vi "RunAcquisition.vi"(8 "error in (no error)":errorcluster, 11 "NIScope in":refnum<class "NIScope.lvclass">) -> (0 "error out":errorcluster, 1 "output cluster":T1, 2 "Waveforms":T3[](array[typedef]), 3 "NIScope out":refnum<class "NIScope.lvclass">)   [LabVIEW 2018, in "ScopePlugins.lvlib" / "NIScope.lvclass"]
doc: "Retrieves data from the instrument(s)."
uses:
  NIScope.lvclass
  F:/Projects/ICDAS/NistPluggableModules/Scope/ScopePlugins/ScopePluginBaseClass/ScopePluginsBase.lvclass
  ScopeShared/Waveform.ctl
  ScopeShared/ScopeData.ctl
  ScopePluginBaseClass/ScopePluginsBase.lvclass/ScopePluginsBase.ctl
  ScopePluginBaseClass/Accessors/Read Channels.vi
  <instrlib>/niScope/Acquire/Fetch/niScope Multi Fetch Cluster.vi
  ScopePlugins.lvlib
  ScopeShared/ScopeShared.lvlib
panel:
  out "Waveform Graph":T2(graph)
  out "Absolute":dbl[](array[numeric])
  out "Relative":dbl[](array[numeric])
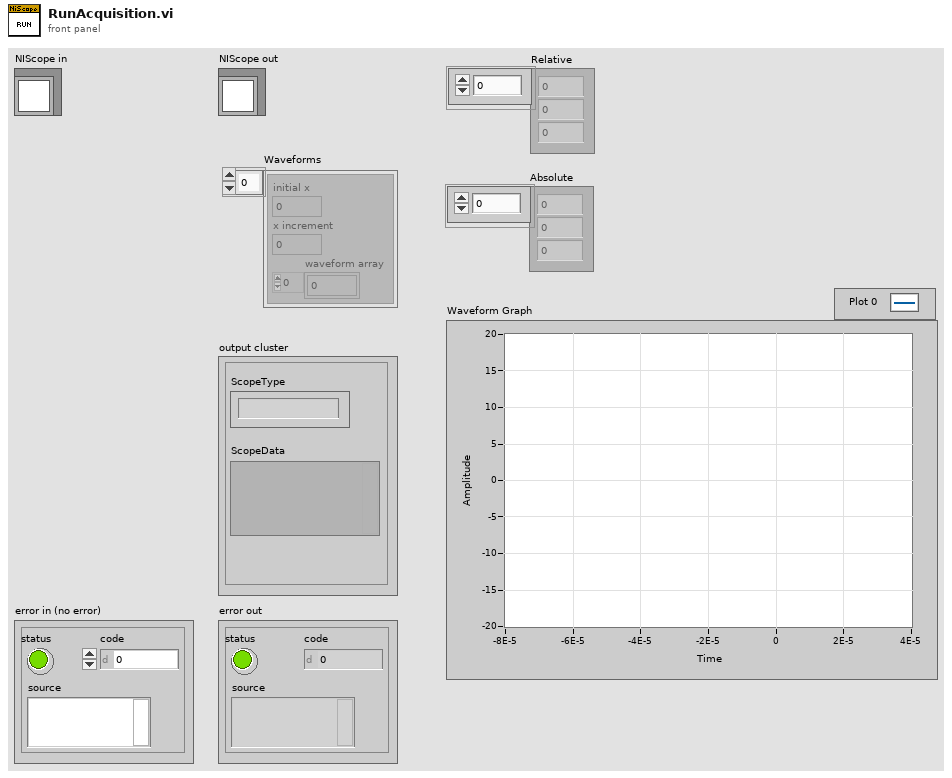
[diagram p1: front panel]
types:
  T1 = typedef "ScopeShared.lvlib/ScopeData.ctl" = cluster{"ScopeType":string, "ScopeData":variant}
  T2 = cluster{"relativeInitialX":dbl, "xIncrement":dbl, "wfm":dbl[]}[]
  T3 = typedef "ScopeShared.lvlib/Waveform.ctl" = cluster{"initial x":dbl, "x increment":dbl, "waveform array":dbl[]}
  T4 = typedef "ScopePlugins.lvlib/ScopePluginsBase.lvclass/InitializationSettings.ctl" = cluster{"Reset":bool, "IdQuery":bool, "AutoConfig":bool, "Options String":string, "Synchronize":bool}
  T5 = typedef "ScopePlugins.lvlib/ScopePluginsBase.lvclass/HorizontalSettings.ctl" = cluster{"Continuous":bool, "EnableAveraging":bool, "Number Averages":i32, "Measurement Timeout":dbl, "Min Record Length":i32, "Min Sample Rate":dbl, "Enforce Realtime":bool, "Sampling Mode ":enum16{"Real Time", "Equivalent Time", "Segment", "Real Time Peak Detect", "Real Time High Resolution", "Peak Detect Segment", "High Resolution Segment"}, "Interpolation":enum16{"No Interpolation", "sin(x)/x", "linear", "1 Point sin(x)/x", "2 Point sin(x)/x", "4 Point sin(x)/x", "8 Point sin(x)/x", "16 Point sin(x)/x"}, "Type":enum16{"Normal", "PeakDetect", "HighRes", "Envelope", "Average"}, "StartTime":dbl, "Time Per Record":dbl, "Number of Points Minimum":i32, "Measurement Name":string, "Measurement RefreshTime (ms)":u32}
  T6 = cluster{"instrument handle":refnum<k15>, string}[]
  T7 = cluster{"actualSamples":i32, "absoluteInitialX":dbl, "relativeInitialX":dbl, "xIncrement":dbl, "offset":dbl, "gain":dbl, "reserved1":dbl, "reserved2":dbl}[]
  T8 = cluster{"relativeInitialX":dbl, "xIncrement":dbl, "wfm":dbl[]}
  T9 = typedef "ScopePlugins.lvlib/ScopePluginsBase.lvclass/ChannelSetting(s).ctl" = cluster{"Number of Channels":i32, "Channel(s)":cluster{"Enabled":bool, "Instrument Handle":string, "Channel Name":string, "Maximum Input Frequency":dbl, "Verticle Settings":cluster{"Vertical Range":dbl, "Vertical Offset":dbl, "Probe Attenuation":dbl, "Vertical Coupling":i32}, "Connected":bool, "Input Impedance":dbl, "IO Type Instrument Handle":refnum<k15>}[]}
  T10 = cluster{"Enabled":bool, "Instrument Handle":string, "Channel Name":string, "Maximum Input Frequency":dbl, "Verticle Settings":cluster{"Vertical Range":dbl, "Vertical Offset":dbl, "Probe Attenuation":dbl, "Vertical Coupling":i32}, "Connected":bool, "Input Impedance":dbl, "IO Type Instrument Handle":refnum<k15>}[]
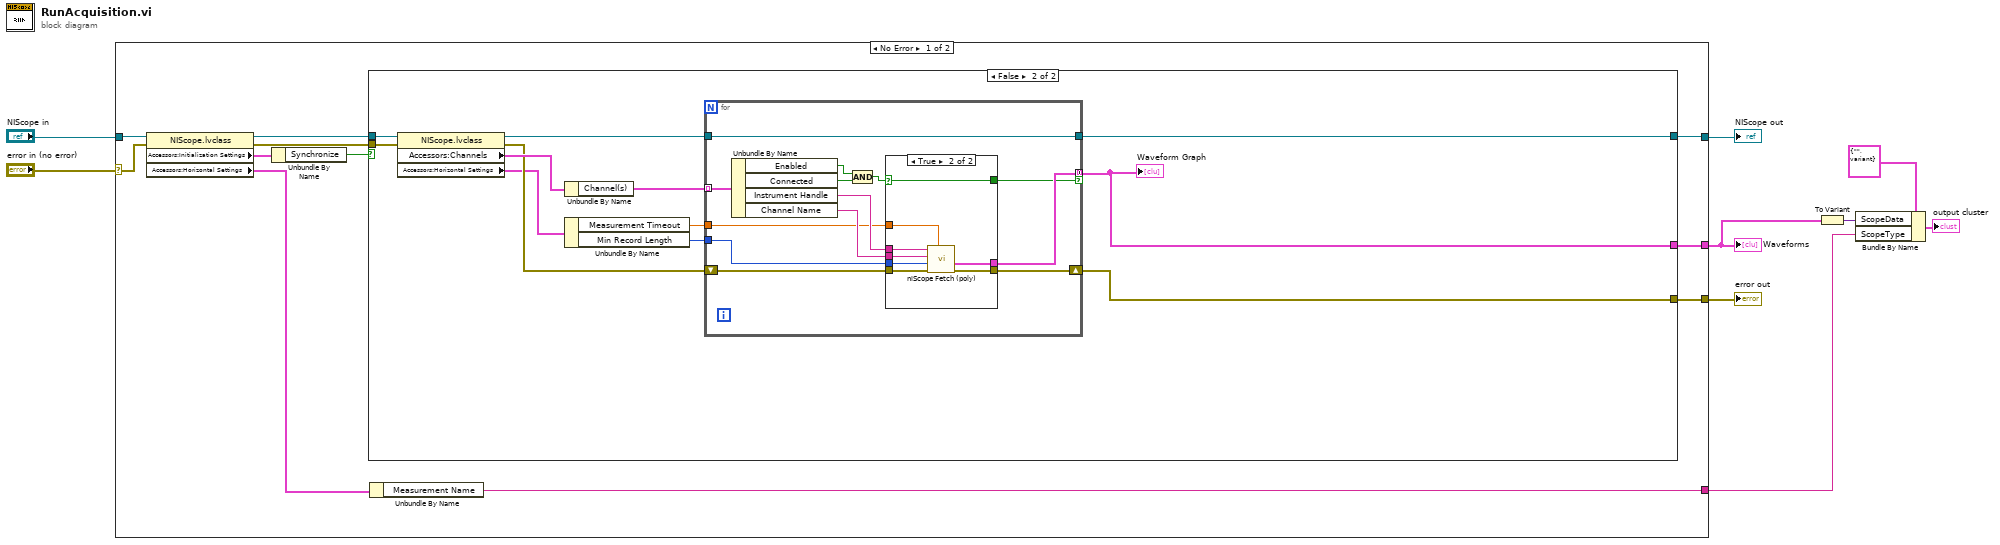
[diagram p0: block diagram]
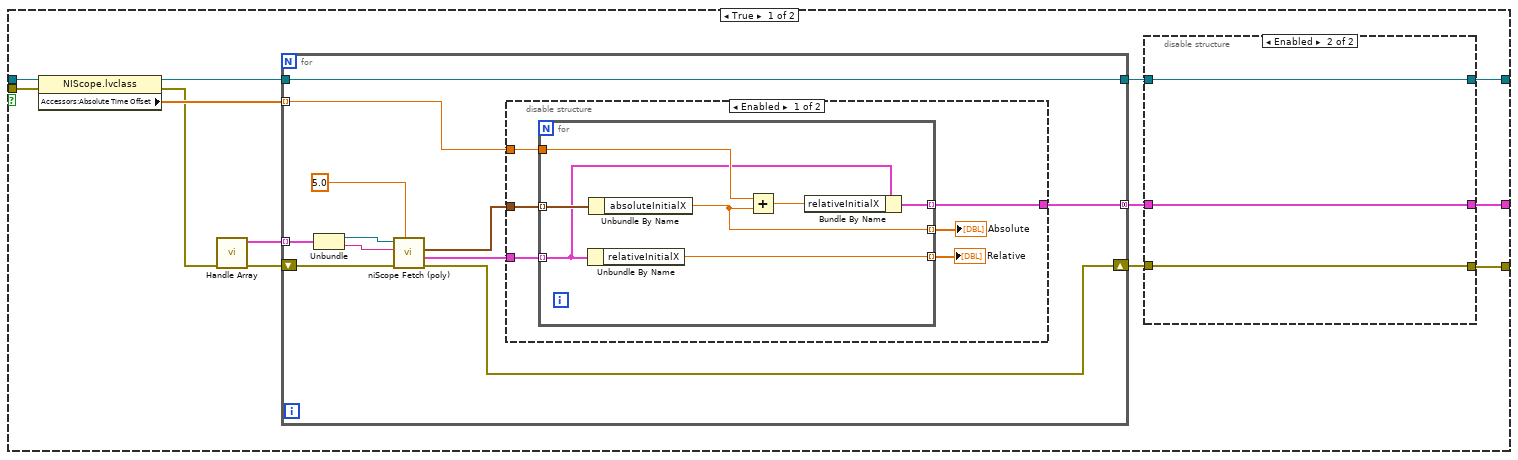
[diagram p2: hidden frame]
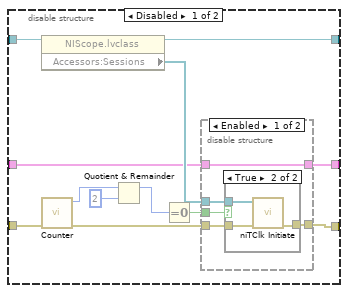
[diagram p4: hidden frame]
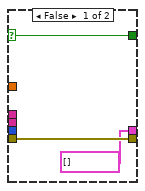
[diagram p7: hidden frame]
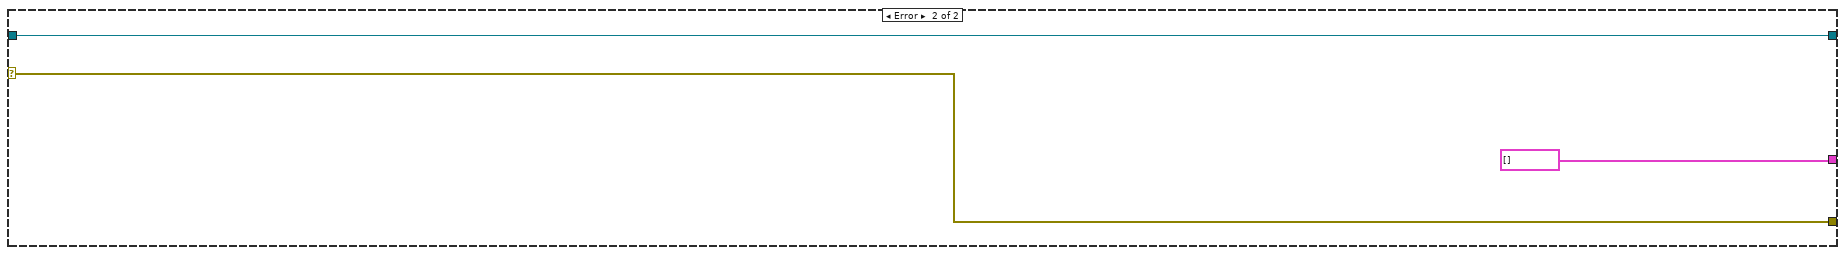
[diagram p8: hidden frame]
diagram:
  n1 = case shown="No Error" "error in (no error)" {
    selector: "error in (no error)" -> [w15 w121]
    tunnel: "NIScope in" -> [w16 w122]
    tunnel: [w19 w122] -> w7
    tunnel: [w18 w121] -> w6
    tunnel: [w20 T2 [] ("waveform")] -> w3
    tunnel: [w10 _] -> w2
    frame No Error {
      n2 = property class="NIScope.lvclass"(reference=w16, error in=w15) -> (reference out=w14:refnum<class "NIScope.lvclass">, error out=w13:errorcluster, "Accessors:Initialization Settings"=w12:T4, "Accessors:Horizontal Settings"=w11:T5)
      n3 = Unbundle By Name(w12) -> ("Synchronize"=w17:bool)
      n4 = case shown="False" w17 {
        tunnel: [w21 w84] -> w20
        tunnel: [w33 w93] -> w19
        tunnel: [w31 w95] -> w18
        tunnel: w13 -> [w27 w91]
        tunnel: w14 -> [w23 w94]
        frame True {
          n5 = property class="NIScope.lvclass"(reference=w23, error in=w27) -> (reference out=w25:refnum<class "NIScope.lvclass">, error out=w26:errorcluster, "Accessors:Absolute Time Offset"=w28:dbl[])
          n6 = call "Handle Array.vi"("error in (no error)"=w26) -> ("error out"=w29:errorcluster, "Array Handles"=w30:T6)  [unwired: 9 in]
          n7 = for {
            tunnel: [w42] -> w22 mode=concatenating
            shift-right: [w34] -> w32
            shift-left: w29 -> [w43]
            tunnel: w30 -> [w40] mode=indexing
            tunnel: w28 -> [w36] mode=indexing
            tunnel: w25 -> [w35]
            tunnel: [w35] -> w24
            n8 = Unbundle(w40) -> ("instrument handle"=w39:refnum<k15>, w38:string)
            n9 = call-poly <instrlib>:"niScope Fetch (poly).vi"("timeout"=5.0, "error in"=w43, "channels"=w38, "instrument handle"=w39) -> ("error out"=w34:errorcluster, "waveform"=w41:T2, "wfm info"=w37:T7)  [unwired: 4 in, 1 out]
            n10 = disable-structure shown="Enabled" {
              disable-tunnel: [w50 w58] -> w42
              disable-tunnel: w41 -> [w49 w58]
              disable-tunnel: w37 -> [w48 _]
              disable-tunnel: w36 -> [w47 _]
              frame Enabled {
                n11 = for {
                  tunnel: w49 -> [w54] mode=indexing
                  tunnel: [w57] -> w50 mode=indexing
                  tunnel: w48 -> [w56] mode=indexing
                  tunnel: w47 -> [w55]
                  tunnel: [w51] -> w46 mode=indexing
                  tunnel: [w53] -> w45 mode=indexing
                  n12 = Unbundle By Name(w54) -> ("relativeInitialX"=w51:dbl)
                  n13 = Unbundle By Name(w56) -> ("absoluteInitialX"=w53:dbl)
                  n14 = Add(x=w55, y=w53) -> (x+y=w52:dbl)
                  n15 = Bundle By Name(cluster=w54, "relativeInitialX"=w52) -> (w57:T8)
                }
                "Relative" <- w46
                "Absolute" <- w45
              }
              frame Disabled {
              }
            }
          }
          n16 = disable-structure shown="Enabled" {
            disable-tunnel: [w70 w83] -> w33
            disable-tunnel: w32 -> [w68 w82]
            disable-tunnel: [w66 w82] -> w31
            disable-tunnel: w24 -> [w61 w83]
            disable-tunnel: w22 -> [w60 w81]
            disable-tunnel: [w59 w81] -> w21
            frame Disabled {
              n17 = property class="NIScope.lvclass"(reference=w61) -> (reference out=w70:refnum<class "NIScope.lvclass">, "Accessors:Sessions"=w69:refnum<k20>[])  [unwired: 1 in, 1 out]
              n18 = call "Counter.vi"("error in (no error)"=w68) -> ("error out"=w67:errorcluster, "Counter Out"=w62:i32)  [unwired: 9 in]
              n19 = Quotient & Remainder(x=w62, y=2) -> (x-y*floor(x/y)=w63:i32)  [unwired: 1 out]
              n20 = Equal To 0?(x=w63) -> (x = 0?=w64:bool)
              n21 = disable-structure shown="Enabled" {
                disable-tunnel: w69 -> [w75 _]
                disable-tunnel: w67 -> [w74 w80]
                disable-tunnel: [w73 w80] -> w66
                disable-tunnel: w64 -> [w72 _]
                disable-tunnel: w60 -> [w71 _]
                disable-tunnel: [w71 _] -> w59
                frame Enabled {
                  n22 = case shown="True" w72 {
                    tunnel: w75 -> [_ w79]
                    tunnel: w74 -> [w76 w78]
                    tunnel: [w76 w77] -> w73
                    frame False {
                    }
                    frame True {
                      n23 = call <instrlib>:"niTClk Initiate.vi"("error in (no error)"=w78, "sessions"=w79) -> ("error out"=w77:errorcluster)  [unwired: 8 in, 1 out]
                    }
                  }
                }
                frame Disabled {
                }
              }
            }
            frame Enabled {
            }
          }
        }
        frame False {
          n24 = property class="NIScope.lvclass"(reference=w94, error in=w91) -> (reference out=w92:refnum<class "NIScope.lvclass">, error out=w88:errorcluster, "Accessors:Channels"=w90:T9, "Accessors:Horizontal Settings"=w87:T5)
          n25 = Unbundle By Name(w90) -> ("Channel(s)"=w89:T10)
          n26 = Unbundle By Name(w87) -> ("Measurement Timeout"=w85:dbl, "Min Record Length"=w86:i32)
          n27 = for {
            tunnel: [w106] -> w84 mode=concatenating if=w100
            shift-right: [w108] -> w95
            shift-left: w88 -> [w107]
            tunnel: w92 -> [w105]
            tunnel: [w105] -> w93
            tunnel: w89 -> [w104] mode=indexing
            tunnel: w86 -> [w101]
            tunnel: w85 -> [w99]
            n28 = Unbundle By Name(w104) -> ("Enabled"=w96:bool, "Connected"=w97:bool, "Instrument Handle"=w103:string, "Channel Name"=w102:string)
            n29 = And(x=w96, y=w97) -> (x .and. y?=w98:bool)
            n30 = case shown="True" w98 {
              selector: w98 -> [w109 w113]
              tunnel: [w111 w119] -> w108
              tunnel: w107 -> [w111 w118]
              tunnel: [T2 [] ("waveform") w117] -> w106
              tunnel: w103 -> [_ w116]
              tunnel: w102 -> [_ w115]
              tunnel: w101 -> [_ w114]
              tunnel: [w109 w113] -> w100
              tunnel: w99 -> [_ w112]
              frame False {
              }
              frame True {
                n31 = call-poly <instrlib>:"niScope Fetch (poly).vi"("timeout"=w112, "error in"=w118, "numSamples"=w114, "channels"=w115, "instrument handle"=w116) -> ("error out"=w119:errorcluster, "waveform"=w117:T2)  [unwired: 3 in, 2 out]
              }
            }
          }
          "Waveform Graph" <- w84
        }
      }
      n32 = Unbundle By Name(w11) -> ("Measurement Name"=w10:string)
    }
    frame Error {
    }
  }
  "error out" <- w6
  "NIScope out" <- w7
  "Waveforms" <- w3
  n33 = To Variant(anything=w3) -> (Variant=w5:variant)
  n34 = Bundle By Name(cluster=T1 {"ScopeType"="", "ScopeData"=variant} ("ScopeData"), "ScopeData"=w5, "ScopeType"=w2) -> (→"output cluster":T1)
